vi "Firmware.vi"() -> ()   [LabVIEW 2015]
uses:
  <vilib>/Platform/TimedLoop/XDataNode/timing_clust.ctl
  <vilib>/Platform/TimedLoop/XDataNode/nitl_modes.ctl
  <vilib>/Platform/TimedLoop/XDataNode/wakeup.ctl
  <vilib>/rvi/Emulation/niFpgaGetClockAttributes.vi
  <vilib>/rvi/Emulation/niFpgaSctlEmulationGetInTimedLoop.vi
  <vilib>/rvi/Emulation/niFpgaEmulationReportErrorSimple.vi
  <vilib>/rvi/Emulation/niFpgaProcessEmulError.vi
  <vilib>/rvi/Emulation/niFpgaCriticalErrorInLSC.vi
  <vilib>/rvi/occurrence/nirviWaitOnOccurrenceBase.vi
  <vilib>/rvi/eio/common/nirviEmuTemplateMethod_errors.vi
  <vilib>/Platform/TimedLoop/XDataNode/XDataNode.xnode
  <vilib>/eio/EIONode/EIONode.xnode
  <instrlib>/_niInstr/Instruction Framework/v1/FPGA/Top Level Bus/Register Configuration/Register Configuration.lvclass
  <vilib>/Platform/TimedLoop/XDataNode/XDNodeRunTimeDep.lvlib
  <vilib>/NI/PowerElectronicsControl/ScaleAndLimit/Core/ScaleAndLimit.lvlib
  <vilib>/NI/PowerElectronicsControl/ScaleAndLimit/Core/AddressSpace.lvclass
  <instrlib>/_niInstr/FIFO Register Bus/v1/FPGA/niInstr FIFO Register Bus v1 FPGA.lvclass
  <vilib>/NI/PowerElectronicsControl/WaveformAcq/IFw_Addon/FPGA/WaveformAddressSpace.lvclass
panel:
  out "TriggerTimestamp":i32
  out "relativeTimestamp":i32
  in  "ManualTrigger":bool
  in  "fifo reg bus ctrl 0":u32
  out "fifo reg bus status 0":u32
  out "fifo reg bus data 0":u64
  out "SimultaneousAILoopRate":u32
  out "ScaledAI":sgl[](array[numeric])
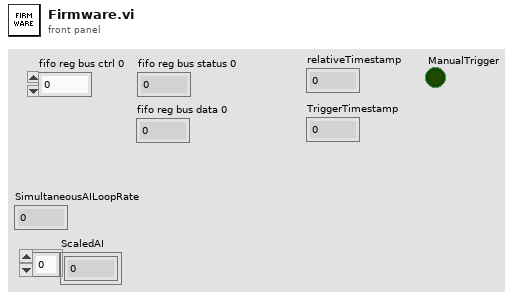
[diagram p1: front panel]
types:
  T1 = typedef "XDNodeRunTimeDep.lvlib/timing_clust.ctl" = cluster{"Expected End [f-1]":u64, "Actual End [f-1]":u64, "Finished Late? [f-1]":bool, "Expected End [i-1]":u64, "Actual End [i-1]":u64, "Finished Late? [i-1]":bool, "Expected Start [i]":u64, "Actual Start [i]":u64, "Expected Start [f]":u64, "Actual Start [f]":u64, "Source Name":string, "Structure Name":string, "Period":i64, "Deadline":i64, "Offset":i64, "Start":i64, "Priority":i32, "Timeout":i32, "Mode":T2, "Wakeup Reason":T3, "Error":errorcluster, "Source Type":string, "Secondary Source Type":string, "Global End Time":u64, "Global Start Time":u64, "Frame Duration":u64, "Iteration Duration":u64, "Assigned CPU":i32, "I/O Scan Engine Mode":u32}
  T2 = typedef "XDNodeRunTimeDep.lvlib/nitl_modes.ctl" = enum32{"No Change", "Process missed periods, maintain original phase", "Discard missed periods, maintain original phase", "Process missed periods, ignore original phase", "Discard missed periods, ignore original phase"}
  T3 = typedef "XDNodeRunTimeDep.lvlib/wakeup.ctl" = enum32{"Normal", "Aborted", "Asynchronous wakeup", "Timing source error", "Timed loop error", "Timeout"}
  T4 = typedef "ScaleAndLimit.lvlib/LimitsRegisters.ctl" = cluster{"HighLimits":refnum<k21>, "LowLimits":refnum<k21>, "ClearLimits":refnum<k21>, "LimitsFlag":refnum<k21>}
  T5 = typedef "ScaleAndLimit.lvlib/ConfigRegisters.ctl" = cluster{"LimitsEnabled":refnum<k21>, "UnscaledHighLimit":refnum<k21>, "UnscaledLowLimit":refnum<k21>, "B":refnum<k21>, "M":refnum<k21>}
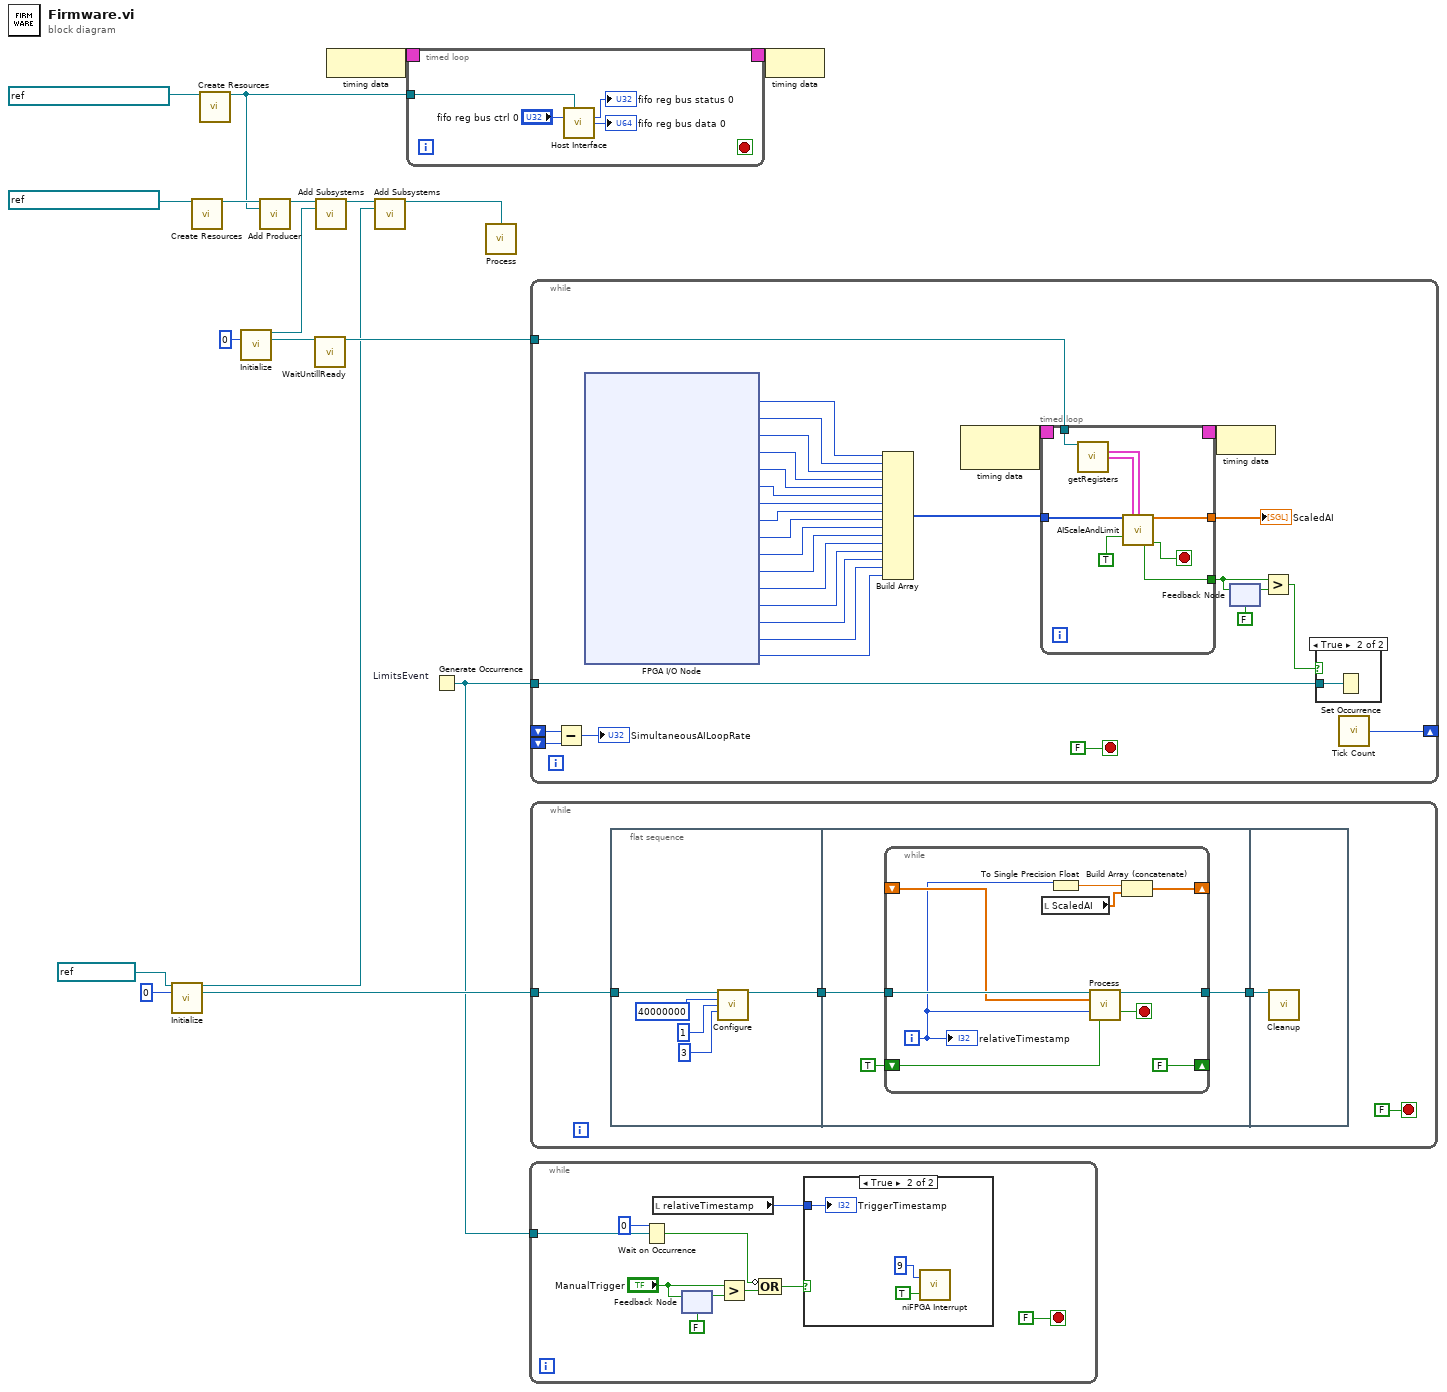
[diagram p0: block diagram]
diagram:
  n1 = call <vilib>:"Initialize.vi"("DMA FIFO"=refnum<k21> "DataSGL0" ("FIFO Out"), "instance"=u8 0) -> ("subsystem"=w2:refnum<class "Single Address Space Collection.lvclass">, "AddressSpace"=w5:refnum<class "WaveformAddressSpace.lvclass">)  [unwired: 12 in]
  n2 = call <instrlib>:"Create Resources.vi"("register clock"=refnum<k21> "40 MHz Onboard Clock") -> ("register configuration"=w16:refnum<class "Register Configuration.lvclass">)  [unwired: 14 in]
  n3 = call <instrlib>:"Create Resources.vi"("instruction fifo"=refnum<k21> "reg.host instruction fifo 0") -> ("fifo register bus"=w8:refnum<class "niInstr FIFO Register Bus v1 FPGA.lvclass">)  [unwired: 14 in]
  n4 = call <vilib>:"Initialize.vi"("instance"=u8 0) -> ("subsystem"=w13:refnum<class "Single Address Space Collection.lvclass">, "AddressSpace"=w11:refnum<class "AddressSpace.lvclass">)  [unwired: 13 in]
  n5 = call <instrlib>:"Add Producer.vi"("register configuration in"=w16, "instruction producer"=w8) -> ("register configuration out"=w14:refnum<class "Register Configuration.lvclass">)  [unwired: 13 in]
  n6 = call <vilib>:"WaitUntillReady.vi"("AddressSpace in"=w11) -> ("AddressSpace out"=w10:refnum<class "AddressSpace.lvclass">)  [unwired: 14 in]
  n7 = call <instrlib>:"Add Subsystems.vi"("register configuration in"=w14, "subsystems"=w13) -> ("register configuration out"=w4:refnum<class "Register Configuration.lvclass">)  [unwired: 13 in]
  n8 = node-c288() -> (w18:T1)
  n9 = call <instrlib>:"Add Subsystems.vi"("register configuration in"=w4, "subsystems"=w2) -> ("register configuration out"=w3:refnum<class "Register Configuration.lvclass">)  [unwired: 13 in]
  n10 = timed-loop {
    timing: w18 -> [_]
    timing-out: [_] -> w17
    tunnel: w8 -> [w22]
    stop <- _ stop-if-true
    n11 = call <instrlib>:"Host Interface.vi"("fifo register bus"=w22, "fifo reg bus ctrl 0"="fifo reg bus ctrl 0") -> ("fifo reg bus status 0"=→"fifo reg bus status 0":u32, "fifo reg bus data 0"=→"fifo reg bus data 0":u64)  [unwired: 12 in]
  }
  n12 = Generate Occurrence "LimitsEvent"() -> (w1:refnum<k4>)
  n13 = call <instrlib>:"Process.vi"("register configuration"=w3) -> ()  [unwired: 15 in]
  n14 = while {
    tunnel: w1 -> [w34]
    stop <- FALSE stop-if-true
    n15 = Wait on Occurrence(2:w34, 3:0 ("ms timeout (-1)")) -> (0:w28:bool)  [unwired: 1 in]
    n16 = local read "relativeTimestamp"() -> (w25:i32)
    n17 = feedback-in #1("ManualTrigger") -> ()
    n18 = feedback #1(FALSE ("ManualTrigger")) -> (w30:bool)
    n19 = Greater?(x="ManualTrigger", y=w30) -> (0:w31:bool)
    n20 = Compound Arithmetic op=OR(invert w28, w31) -> (w27:bool)
    n21 = case shown="True" w27 {
      tunnel: w25 -> [_ w35]
      frame False {
      }
      frame True {
        n22 = call <vilib>:"niFPGA Interrupt.vi"("Wait Until Cleared (F)"=TRUE, "IRQ Number (0)"=u8 9) -> ()  [unwired: 1 in]
        "TriggerTimestamp" <- w35
      }
    }
  }
  n23 = while {
    shift-right: [w67] -> _
    shift-left: _ -> [w66]
    shift-left: _ -> [w65]
    tunnel: w10 -> [w45]
    tunnel: w1 -> [w39]
    stop <- FALSE stop-if-true
    n24 = Subtract(x=w66, y=w65) -> (x-y=→"SimultaneousAILoopRate":u32)
    n25 = xnode "FPGA I/O Node"() -> ("RMC/Simultaneous/AI0"=w63:i16, "RMC/Simultaneous/AI1"=w62:i16, "RMC/Simultaneous/AI2"=w61:i16, "RMC/Simultaneous/AI3"=w60:i16, "RMC/Simultaneous/AI4"=w59:i16, "RMC/Simultaneous/AI5"=w58:i16, "RMC/Simultaneous/AI6"=w57:i16, "RMC/Simultaneous/AI7"=w56:i16, "RMC/Simultaneous/AI8"=w55:i16, "RMC/Simultaneous/AI9"=w54:i16, "RMC/Simultaneous/AI10"=w53:i16, "RMC/Simultaneous/AI11"=w52:i16, "RMC/Simultaneous/AI12"=w51:i16, "RMC/Simultaneous/AI13"=w50:i16, "RMC/Simultaneous/AI14"=w49:i16, "RMC/Simultaneous/AI15"=w43:i16)  [unwired: 16 in, 16 out]
    n26 = Build Array(w63, w62, w61, w60, w59, w58, w57, w56, w55, w54, w53, w52, w51, w50, w49, w43) -> (w44:i16[])
    n27 = node-c288() -> (w48:T1)  [unwired: 1 in]
    n28 = timed-loop {
      timing: w48 -> [_]
      timing-out: [_] -> w47
      tunnel: w44 -> [w77]
      tunnel: [w75] -> w46
      tunnel: w45 -> [w73]
      tunnel: [w70] -> w42
      stop <- w74 stop-if-true
      n29 = call <vilib>:"getRegisters.vi"("AddressSpace in"=w73) -> ("LimitsRegisters"=w71:T4, "ConfigRegisters"=w72:T5)  [unwired: 12 in, 1 out]
      n30 = call <vilib>:"AIScaleAndLimit.vi"("UnscaledAI"=w77, "ConfigRegisters"=w72, "LimitsRegisters"=w71, "input valid"=TRUE) -> ("ScaledAI"=w75:sgl[], "LimitsFlag"=w70:bool, "output valid"=w74:bool)  [unwired: 6 in, 3 out]
    }
    "ScaledAI" <- w46
    n31 = node-c288(w47) -> ()
    n32 = feedback-in #2(w42) -> ()
    n33 = feedback #2(FALSE ("LimitsFlag")) -> (w40:bool)
    n34 = Greater?(x=w42, y=w40) -> (0:w38:bool)
    n35 = case shown="True" w38 {
      tunnel: w39 -> [_ w69]
      frame False {
      }
      frame True {
        n36 = Set Occurrence(w69) -> ()
      }
    }
    n37 = call "Tick Count"() -> ("Tick Count(Ticks)"=w67:u32)
  }
  n38 = while {
    tunnel: w5 -> [w82]
    stop <- FALSE stop-if-true
    n39 = flat-sequence {
      tunnel: [w86] -> w84
      tunnel: w82 -> [w87]
      tunnel: w84 -> [w93]
      tunnel: [w92] -> w83
      tunnel: w83 -> [w104]
      frame #0 {
        n40 = call <vilib>:"Configure.vi"("WaveformAddressSpace in"=w87, "oclk_freq"=u32 40000000, "oclk_mult"=u32 1, "UnderflowMargin"=u32 3 ("y")) -> ("WaveformAddressSpace out"=w86:refnum<class "WaveformAddressSpace.lvclass">)  [unwired: 11 in]
      }
      frame #1 {
        n41 = while {
          shift-right: [w102] -> _
          shift-left: _ -> [w96]
          shift-right: [FALSE] -> _
          shift-left: TRUE -> [w98]
          tunnel: w93 -> [w100]
          tunnel: [w99] -> w92
          i -> [w95]
          stop <- w101 stop-if-true
          n42 = local read "ScaledAI"() -> (w97:sgl[])
          n43 = To Single Precision Float(number=w95) -> (single precision float=w94:sgl)
          n44 = call <instrlib>:"Process.vi"("WaveformAddressSpace in"=w100, "Data"=w96, "Iteration"=w95, "FirstIteration"=w98) -> ("WaveformAddressSpace out"=w99:refnum<class "WaveformAddressSpace.lvclass">, "stop"=w101:bool)  [unwired: 8 in, 2 out]
          n45 = Build Array (concatenate)(w94, w97) -> (w102:sgl[])
          "relativeTimestamp" <- w95
        }
      }
      frame #2 {
        n46 = call <vilib>:"Cleanup.vi"("WaveformAddressSpace in"=w104) -> ()  [unwired: 14 in, 1 out]
      }
    }
  }
  n47 = node-c288(w17) -> ()
